vi "Escape Reserve Word.vi"(8 "error in (no error)":errorcluster, 10 "Input Name":string, 11 "DBMS Specific in":refnum<class "DBMS Specific.lvclass">) -> (0 "error out":errorcluster, 2 "Escaped Name":string, 3 "DBMS Specific out":refnum<class "DBMS Specific.lvclass">)   [LabVIEW 2020, in "ADODB.lvlib" / "DBMS Specific.lvclass"]
uses:
  DBMS Specific.lvclass
panel:
  # "The method takes an input name and checks it against a reserve word list. \n-If the name is reserved, this method attempts to add escape characters to allow for a valid SQL query\n-If escaping the word is not possible, this method returns an error\n-If the the name is not reserved, the method returns a copy of the name"
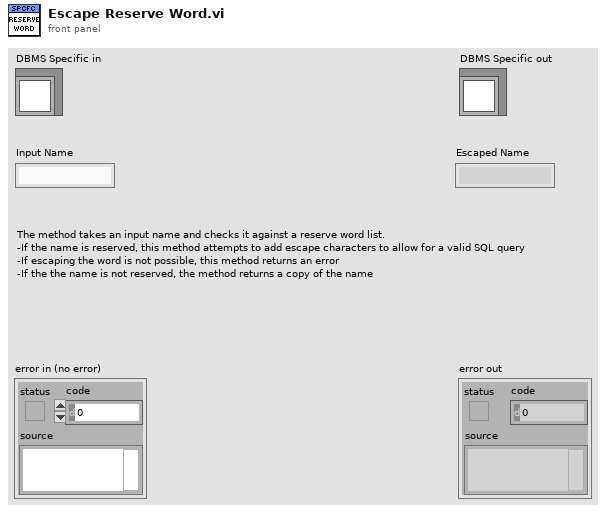
[diagram p1: front panel]
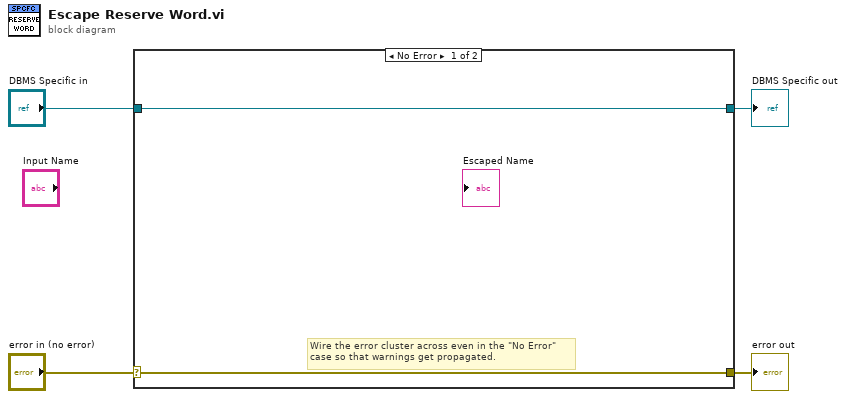
[diagram p0: block diagram]
diagram:
  n1 = case shown="No Error" "error in (no error)" {
    selector: "error in (no error)" -> [w5 w8]
    tunnel: [w5 w8] -> w3
    tunnel: [w6 w7] -> w1
    tunnel: "DBMS Specific in" -> [w6 w7]
    frame No Error {
      # "Wire the error cluster across even in the \"No Error\"\ncase so that warnings get propagated."
    }
    frame Error {
    }
  }
  "error out" <- w3
  "DBMS Specific out" <- w1
